vi "CH0_write_byte_data_into_mem_no_g_Rev01.vi"(0 "MB data":u8, 1 "UB data":u8, 3 "USB Interface Name":refnum<visa-resource-name>="COM3", 4 "HB data":u8, 5 "LB data":u8, 6 "MB address":string, 7 "HB address":string, 9 "WRITE DATA":bool, 10 "Input buffer size":u32=16384, 11 "LB address":string, 12 "UB address":string, 13 "error in (no error)":errorcluster) -> (14 "MB data string":string, 15 "UB data string":string, 17 "error out":errorcluster, 18 "HB data string":string, 19 "LB data string":string)   [LabVIEW 2012]
panel:
  out "T command Bytes sent 4":dbl
  out "T command Bytes sent 3":dbl
  out "T command Bytes sent 2":dbl
  out "T command Bytes sent":dbl
  out "First 'T' Number of bytes written":dbl
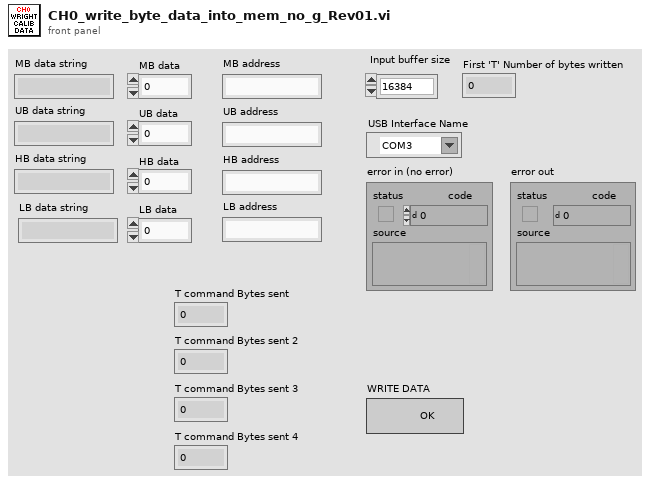
[diagram p1: front panel]
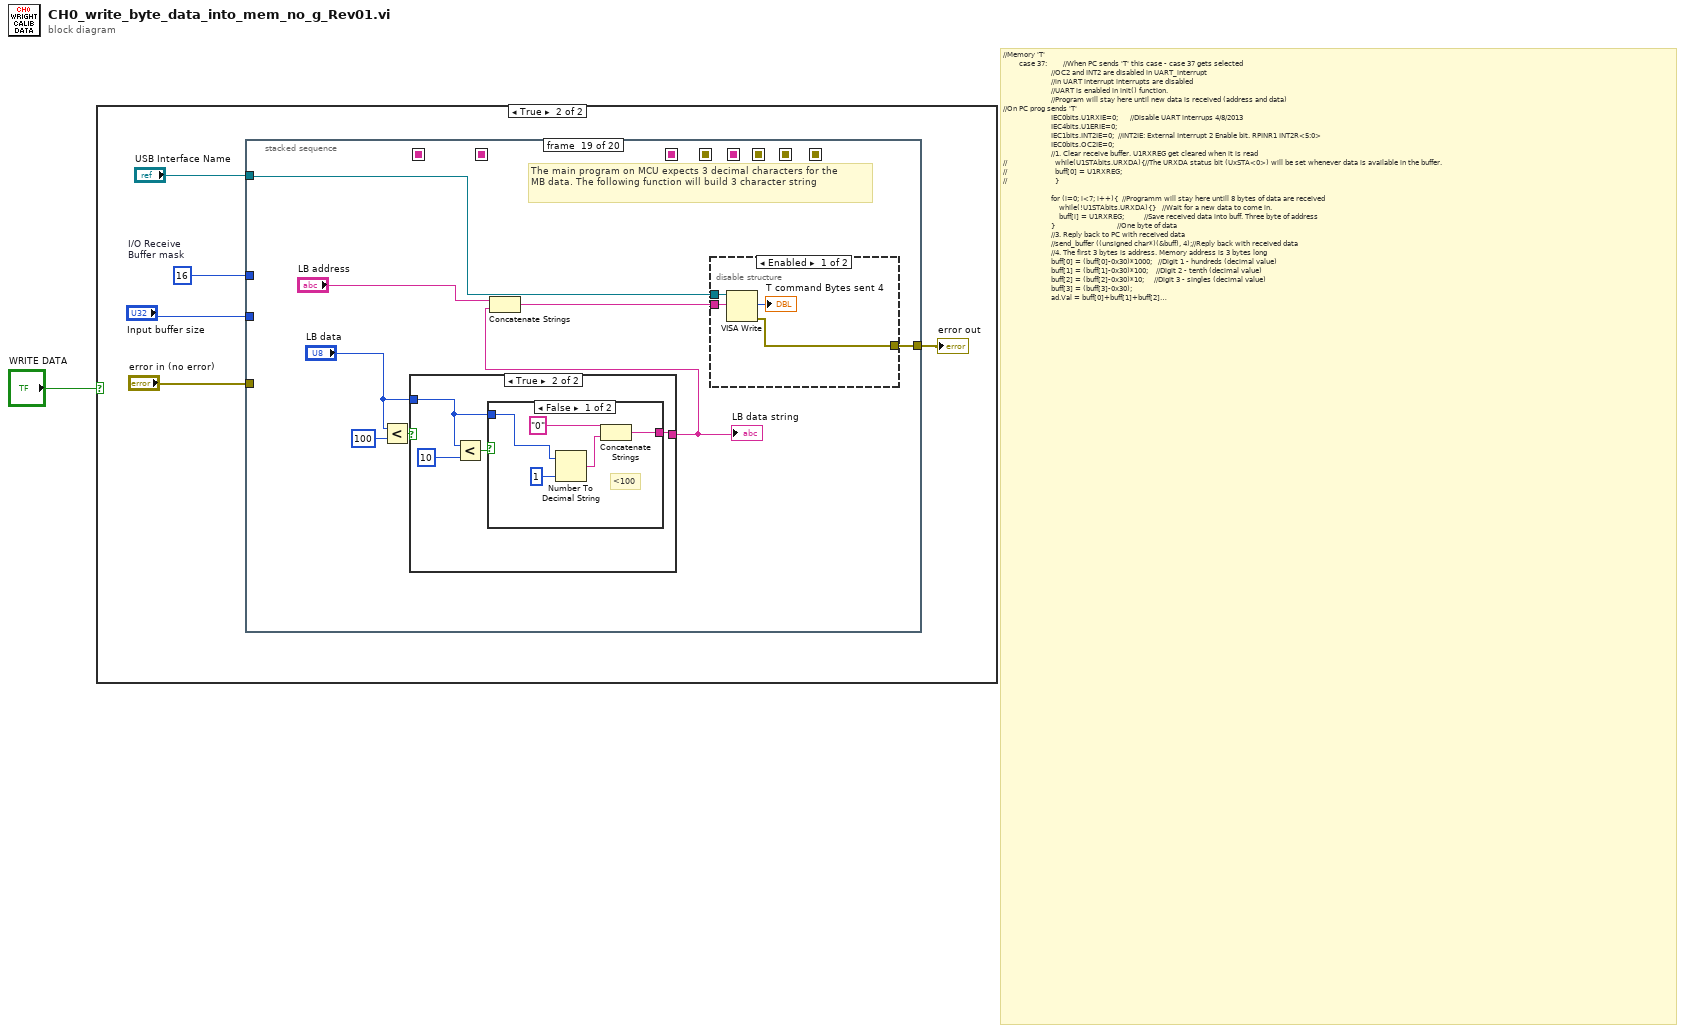
[diagram p0: block diagram]
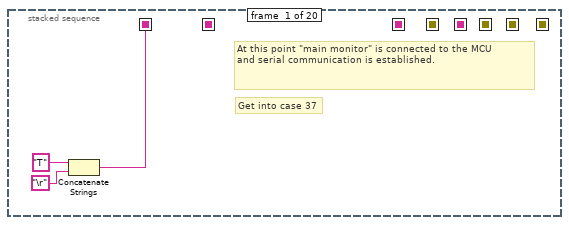
[diagram p3: hidden frame]
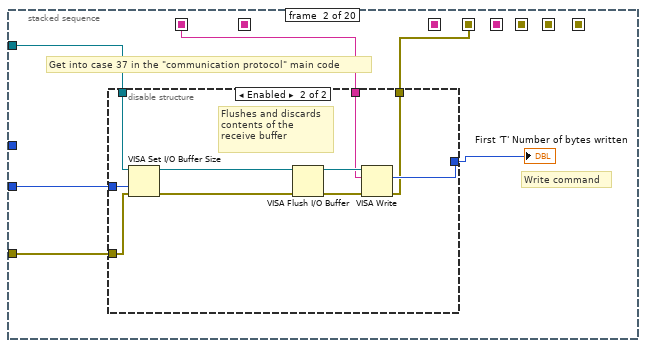
[diagram p4: hidden frame]
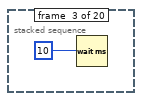
[diagram p6: hidden frame]
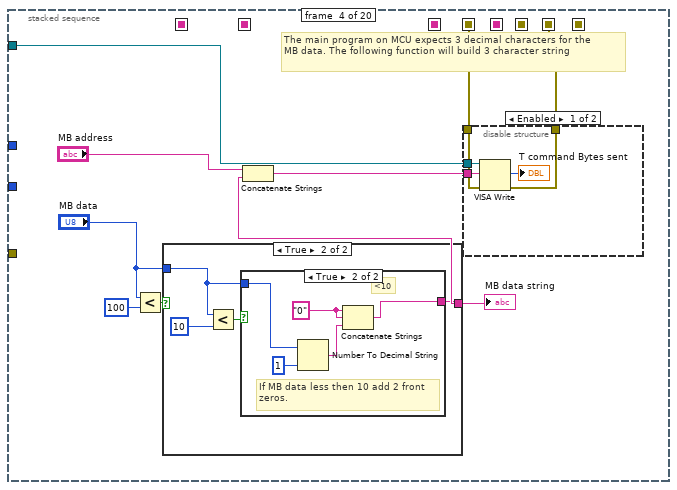
[diagram p7: hidden frame]
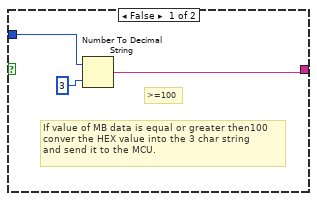
[diagram p8: hidden frame]
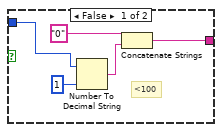
[diagram p9: hidden frame]
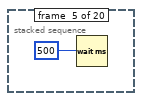
[diagram p11: hidden frame]
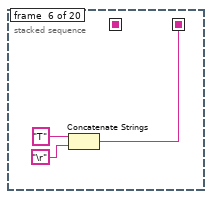
[diagram p12: hidden frame]
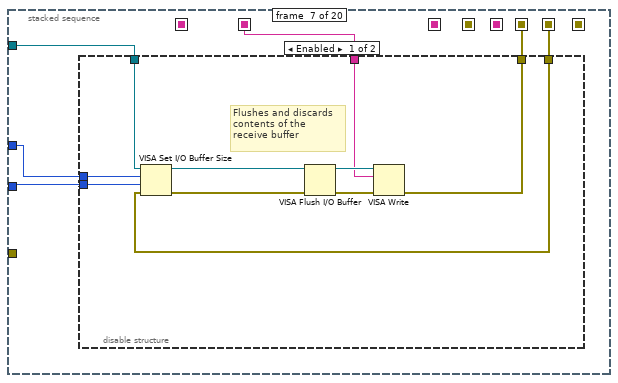
[diagram p13: hidden frame]
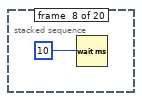
[diagram p15: hidden frame]
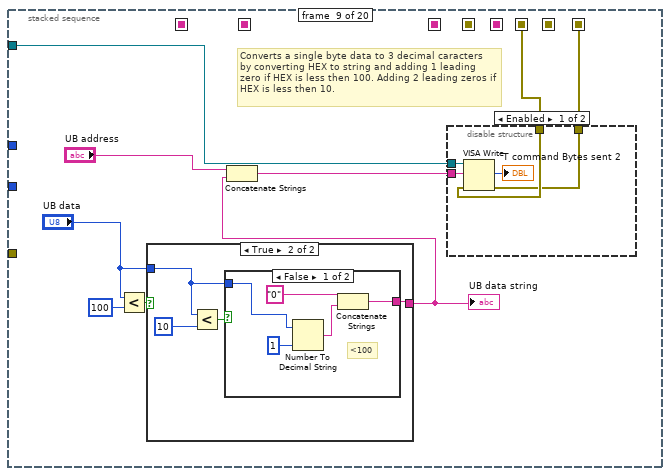
[diagram p16: hidden frame]
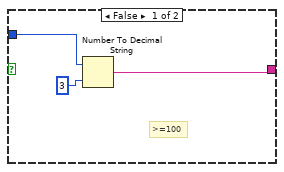
[diagram p17: hidden frame]
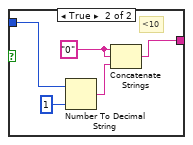
[diagram p18: hidden frame]
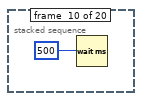
[diagram p20: hidden frame]
diagram:
  # "//Memory 'T'\n        case 37:        //When PC sends 'T' this case - case 37 gets selected\n                        //OC2 and INT2 are disabled in UART_interrupt\n                        //in UART interrupt interrupts are disabled\n                        //UART is enabled in init() function.\n                        //Program will stay here until new data is received (address and data)\n//On PC prog sends 'T'\n                        IEC0bits.U1RXIE=0;      //Disable UART interrups 4/8/2013\n                        IEC4bits.U1ERIE=0;\n                        IEC1bits.INT2IE=0;  //INT2IE: External Interrupt 2 Enable bit. RPINR1 INT2R<5:0>\n                        IEC0bits.OC2IE=0;\n                        //1. Clear receive buffer. U1RXREG get cleared when it is read\n//                        while(U1STAbits.URXDA){//The URXDA status bit (UxSTA<0>) will be set whenever data is available in the buffer.\n//                        buff[0] = U1RXREG;\n//                        }\n\n                        for (i=0; i<7; i++){  //Programm will stay here untill 8 bytes of data are received\n                            while(!U1STAbits.URXDA){}   //Wait for a new data to come in.\n                            buff[i] = U1RXREG;          //Save received data into buff. Three byte of address\n                        }                               //One byte of data\n                        //3. Reply back to PC with received data\n                        //send_buffer ((unsigned char*)(&buff), 4);//Reply back with received data\n                        //4. The first 3 bytes is address. Memory address is 3 bytes long\n                        buff[0] = (buff[0]-0x30)*1000;   //Digit 1 - hundreds (decimal value)\n                        buff[1] = (buff[1]-0x30)*100;    //Digit 2 - tenth (decimal value)\n                        buff[2] = (buff[2]-0x30)*10;     //Digit 3 - singles (decimal value)\n                        buff[3] = (buff[3]-0x30);\n                        ad.Val = buff[0]+buff[1]+buff[2]+buff[3];\n//                        send_char((char) ad.byte.MB);\n//                        send_char((char) ad.byte.UB);\n//                        send_char((char) ad.byte.HB);\n//                        send_char((char) ad.byte.LB); \n                        //5. The last 3 bytes are data\n                        buff[4] = buff[4]-0x30;//Load data. Byte number 4 is the data byte\n                        buff[5] = buff[5]-0x30;\n                        buff[6] = buff[6]-0x30;\n                        data = buff[4]*100+buff[5]*10+buff[6]; //Decimal value of 3 char digits\n                        //send_buffer ((unsigned char*)(&ad), 3);//Send back the received address\n                        //Erase byte by writing FFH into the address\n                        DF_WriteProtectDisable();   //Enable write to memory\n                        DF_IsBusy();                //Wait until the operation is done\n                        DF_WriteByte(ad.Val, data); //Write data into ad\n                        DF_IsBusy();\n                        DF_WriteDisable();          //Disable write\n                        DF_IsBusy();                        \n                        data=DF_ReadByte(ad.Val);     //4/22/13 return BYTE data\n//                       send_char((char) data);              //Read the memory location and reply with previously sent data\n//                        //Memory address for sign\n//                        buff[7] = (buff[7]-0x30)*1000;   //Digit 1 - hundreds (decimal value)\n//                        buff[8] = (buff[8]-0x30)*100;    //Digit 2 - tenth (decimal value)\n//                        buff[9] = (buff[9]-0x30)*10;     //Digit 3 - singles (decimal value)\n//                        buff[10] = (buff[10]-0x30);\n//                        ad.Val = buff[7]+buff[8]+buff[9]+buff[10];\n//                        //sign\n//                        sgn = buff[11];//<12\n                        \n                        selection = 1;\n                        rx_function=0; //4/11/13\n                        IEC0bits.U1RXIE=1;      //Reinable UART interrups\n                        IEC4bits.U1ERIE=1;                        \n                        IEC1bits.INT2IE=1;  //INT2IE: External Interrupt 2 Enable bit. RPINR1 INT2R<5:0>\n                        IEC0bits.OC2IE=1;\n                        \n\n            break;"
  n1 = case shown="True" "WRITE DATA" {
    frame False {
    }
    frame True {
      w4 = u16 16  # I/O Receive Buffer mask
      n2 = stacked-sequence {
        seq-local: [w7 _ _ _ _ _ _ _ _ _ _ _ _ _ _ _ _ _ _ _] -> [_ w12 _ _ _ _ _ _ _ _ _ _ _ _ _ _ _ _ _ _]
        seq-local: [_ _ _ _ _ w59 _ _ _ _ _ _ _ _ _ _ _ _ _ _] -> [_ _ _ _ _ _ w64 _ _ _ _ _ _ _ _ _ _ _ _ _]
        seq-local: [_ _ _ _ _ _ _ _ _ _ w111 _ _ _ _ _ _ _ _ _] -> [_ _ _ _ _ _ _ _ _ _ _ w115 _ _ _ _ _ _ _ _]
        seq-local: [_ _ _ _ _ _ _ _ _ _ _ _ _ _ _ w157 _ _ _ _] -> [_ _ _ _ _ _ _ _ _ _ _ _ _ _ _ _ w160 _ _ _]
        seq-local: [_ w10 _ _ _ _ _ _ _ _ _ _ _ _ _ _ _ _ _ _] -> [_ _ _ w28 _ _ _ _ _ _ _ _ _ _ _ _ _ _ _ _]
        seq-local: [_ _ _ w27 _ _ _ _ _ _ _ _ _ _ _ _ _ _ _ _] -> [_ _ _ _ _ _ w63 _ _ _ _ _ _ _ _ _ _ _ _ _]
        seq-local: [_ _ _ _ _ _ w62 _ _ _ _ _ _ _ _ _ _ _ _ _] -> [_ _ _ _ _ _ _ _ w80 _ _ _ _ _ _ _ _ _ _ _]
        seq-local: [_ _ _ _ _ _ _ _ w79 _ _ _ _ _ _ _ _ _ _ _] -> [_ _ _ _ _ _ _ _ _ _ _ w114 _ _ _ _ _ _ _ _]
        tunnel: "USB Interface Name" -> [_ w15 _ w34 _ _ w67 _ w82 _ _ w118 _ w130 _ _ w164 _ w178 _]
        tunnel: "error in (no error)" -> [_ w14 _ _ _ _ _ _ _ _ _ _ _ _ _ _ w162 _ _ _]
        tunnel: "Input buffer size" -> [_ w13 _ _ _ _ w66 _ _ _ _ w116 _ _ _ _ w163 _ _ _]
        tunnel: w4 -> [_ _ _ _ _ _ w65 _ _ _ _ w117 _ _ _ _ w161 _ _ _]
        tunnel: [_ _ _ _ _ _ _ _ _ _ _ _ _ _ _ _ _ _ w176 _] -> w3
        frame #0 {
          # "At this point \"main monitor\" is connected to the MCU\nand serial communication is established."
          # "Get into case 37"
          n3 = Concatenate Strings("T", "\r") -> (w7:string)
        }
        frame #1 {
          # "Get into case 37 in the \"communication protocol\" main code"
          # "Write command"
          n4 = disable-structure shown="Enabled" {
            disable-tunnel: w13 -> [_ w21]
            disable-tunnel: w12 -> [_ w20]
            disable-tunnel: w15 -> [_ w19]
            disable-tunnel: w14 -> [_ w18]
            disable-tunnel: [_ w17] -> w11
            disable-tunnel: [_ w16] -> w10
            frame Disabled {
            }
            frame Enabled {
              # "Flushes and discards \ncontents of the \nreceive buffer"
              n5 = VISA Set I/O Buffer Size(VISA resource name=w19, size (4096)=w21, error in (no error)=w18) -> (VISA resource name out=w23:refnum<visa-resource-name>, error out=w22:errorcluster)  [unwired: 1 in]
              n6 = VISA Flush I/O Buffer(VISA resource name=w23, error in (no error)=w22) -> (VISA resource name out=w25:refnum<visa-resource-name>, error out=w24:errorcluster)  [unwired: 1 in]
              n7 = VISA Write(VISA resource name=w25, write buffer=w20, error in (no error)=w24) -> (return count=w17:u32, error out=w16:errorcluster)  [unwired: 1 out]
            }
          }
          "First 'T' Number of bytes written" <- w11
        }
        frame #2 {
          n8 = Wait (ms)(milliseconds to wait=10) -> ()  [unwired: 1 out]
        }
        frame #3 {
          # "The main program on MCU expects 3 decimal characters for the \nMB data. The following function will build 3 character string"
          n9 = Less?(x="MB data", y=100) -> (x < y?=w32:bool)
          n10 = case shown="True" w32 {
            tunnel: [w38 w39] -> w29
            tunnel: "MB data" -> [w36 w40]
            frame False {
              # "If value of MB data is equal or greater then100\nconver the HEX value into the 3 char string \nand send it to the MCU."
              # ">=100"
              n11 = Number To Decimal String(number=w36, width (-)=3) -> (decimal integer string=w38:string)
            }
            frame True {
              n12 = Less?(x=w40, y=10) -> (x < y?=w42:bool)
              n13 = case shown="True" w42 {
                tunnel: w40 -> [w44 w48]
                tunnel: [w43 w49] -> w39
                frame False {
                  # "<100"
                  n14 = Number To Decimal String(number=w44, width (-)=1) -> (decimal integer string=w45:string)
                  n15 = Concatenate Strings("0", w45) -> (w43:string)
                }
                frame True {
                  w50 = "0"
                  # "If MB data less then 10 add 2 front\nzeros."
                  # "<10"
                  n16 = Number To Decimal String(number=w48, width (-)=1) -> (decimal integer string=w51:string)
                  n17 = Concatenate Strings(w50, w50, w51) -> (w49:string)
                }
              }
            }
          }
          "MB data string" <- w29
          n18 = Concatenate Strings("MB address", w29) -> (w35:string)
          n19 = disable-structure shown="Enabled" {
            disable-tunnel: w35 -> [w56 _]
            disable-tunnel: w34 -> [w55 _]
            disable-tunnel: w28 -> [w54 _]
            disable-tunnel: [w53 _] -> w27
            frame Enabled {
              n20 = VISA Write(VISA resource name=w55, write buffer=w56, error in (no error)=w54) -> (return count=→"T command Bytes sent":u32, error out=w53:errorcluster)  [unwired: 1 out]
            }
            frame Disabled {
            }
          }
        }
        frame #4 {
          n21 = Wait (ms)(milliseconds to wait=500) -> ()  [unwired: 1 out]
        }
        frame #5 {
          n22 = Concatenate Strings("T", "\r") -> (w59:string)
        }
        frame #6 {
          n23 = disable-structure shown="Enabled" {
            disable-tunnel: w67 -> [w73 _]
            disable-tunnel: w66 -> [w72 _]
            disable-tunnel: w65 -> [w71 _]
            disable-tunnel: w64 -> [w70 _]
            disable-tunnel: w63 -> [w69 _]
            disable-tunnel: [w68 _] -> w62
            frame Enabled {
              # "Flushes and discards \ncontents of the \nreceive buffer"
              n24 = VISA Set I/O Buffer Size(VISA resource name=w73, mask (16)=w71, size (4096)=w72, error in (no error)=w69) -> (VISA resource name out=w75:refnum<visa-resource-name>, error out=w74:errorcluster)
              n25 = VISA Flush I/O Buffer(VISA resource name=w75, error in (no error)=w74) -> (VISA resource name out=w77:refnum<visa-resource-name>, error out=w76:errorcluster)  [unwired: 1 in]
              n26 = VISA Write(VISA resource name=w77, write buffer=w70, error in (no error)=w76) -> (error out=w68:errorcluster)  [unwired: 2 out]
            }
            frame Disabled {
            }
          }
        }
        frame #7 {
          n27 = Wait (ms)(milliseconds to wait=10) -> ()  [unwired: 1 out]
        }
        frame #8 {
          # "Converts a single byte data to 3 decimal caracters\nby converting HEX to string and adding 1 leading zero if HEX is less then 100. Adding 2 leading zeros if HEX is less then 10."
          n28 = Less?(x="UB data", y=100) -> (x < y?=w86:bool)
          n29 = case shown="True" w86 {
            tunnel: [w90 w91] -> w83
            tunnel: "UB data" -> [w88 w92]
            frame False {
              # ">=100"
              n30 = Number To Decimal String(number=w88, width (-)=3) -> (decimal integer string=w90:string)
            }
            frame True {
              n31 = Less?(x=w92, y=10) -> (x < y?=w94:bool)
              n32 = case shown="False" w94 {
                tunnel: w92 -> [w96 w100]
                tunnel: [w95 w101] -> w91
                frame False {
                  # "<100"
                  n33 = Number To Decimal String(number=w96, width (-)=1) -> (decimal integer string=w97:string)
                  n34 = Concatenate Strings("0", w97) -> (w95:string)
                }
                frame True {
                  w102 = "0"
                  # "<10"
                  n35 = Number To Decimal String(number=w100, width (-)=1) -> (decimal integer string=w103:string)
                  n36 = Concatenate Strings(w102, w102, w103) -> (w101:string)
                }
              }
            }
          }
          "UB data string" <- w83
          n37 = Concatenate Strings("UB address", w83) -> (w87:string)
          n38 = disable-structure shown="Enabled" {
            disable-tunnel: w87 -> [w108 _]
            disable-tunnel: w82 -> [w107 _]
            disable-tunnel: w80 -> [w106 _]
            disable-tunnel: [w105 _] -> w79
            frame Enabled {
              n39 = VISA Write(VISA resource name=w107, write buffer=w108, error in (no error)=w106) -> (return count=→"T command Bytes sent 2":u32, error out=w105:errorcluster)  [unwired: 1 out]
            }
            frame Disabled {
            }
          }
        }
        frame #9 {
          n40 = Wait (ms)(milliseconds to wait=500) -> ()  [unwired: 1 out]
        }
        frame #10 {
          n41 = Concatenate Strings("T", "\r") -> (w111:string)
        }
        frame #11 {
          n42 = disable-structure shown="Enabled" {
            disable-tunnel: w118 -> [w123 _]
            disable-tunnel: w117 -> [w122 _]
            disable-tunnel: w116 -> [w121 _]
            disable-tunnel: w115 -> [w120 _]
            disable-tunnel: w114 -> [w119 _]
            frame Enabled {
              # "Flushes and discards \ncontents of the \nreceive buffer"
              n43 = VISA Set I/O Buffer Size(VISA resource name=w123, mask (16)=w122, size (4096)=w121, error in (no error)=w119) -> (VISA resource name out=w125:refnum<visa-resource-name>, error out=w124:errorcluster)
              n44 = VISA Flush I/O Buffer(VISA resource name=w125, error in (no error)=w124) -> (VISA resource name out=w127:refnum<visa-resource-name>, error out=w126:errorcluster)  [unwired: 1 in]
              n45 = VISA Write(VISA resource name=w127, write buffer=w120, error in (no error)=w126) -> ()  [unwired: 3 out]
            }
            frame Disabled {
            }
          }
        }
        frame #12 {
          n46 = Wait (ms)(milliseconds to wait=10) -> ()  [unwired: 1 out]
        }
        frame #13 {
          # "Converts a single byte data to 3 decimal caracters\nby converting HEX to string and adding 1 leading zero if HEX is less then 100. Adding 2 leading zeros if HEX is less then 10."
          n47 = Less?(x="HB data", y=100) -> (x < y?=w134:bool)
          n48 = case shown="True" w134 {
            tunnel: [w138 w139] -> w131
            tunnel: "HB data" -> [w136 w140]
            frame False {
              # ">=100"
              n49 = Number To Decimal String(number=w136, width (-)=3) -> (decimal integer string=w138:string)
            }
            frame True {
              n50 = Less?(x=w140, y=10) -> (x < y?=w142:bool)
              n51 = case shown="False" w142 {
                tunnel: w140 -> [w144 w148]
                tunnel: [w143 w149] -> w139
                frame False {
                  # "<100"
                  n52 = Number To Decimal String(number=w144, width (-)=1) -> (decimal integer string=w145:string)
                  n53 = Concatenate Strings("0", w145) -> (w143:string)
                }
                frame True {
                  w150 = "0"
                  # "<10"
                  n54 = Number To Decimal String(number=w148, width (-)=1) -> (decimal integer string=w151:string)
                  n55 = Concatenate Strings(w150, w150, w151) -> (w149:string)
                }
              }
            }
          }
          "HB data string" <- w131
          n56 = Concatenate Strings("HB address", w131) -> (w135:string)
          n57 = disable-structure shown="Enabled" {
            disable-tunnel: w135 -> [w154 _]
            disable-tunnel: w130 -> [w153 _]
            frame Enabled {
              n58 = VISA Write(VISA resource name=w153, write buffer=w154) -> (return count=→"T command Bytes sent 3":u32)  [unwired: 1 in, 2 out]
            }
            frame Disabled {
            }
          }
        }
        frame #14 {
          n59 = Wait (ms)(milliseconds to wait=500) -> ()  [unwired: 1 out]
        }
        frame #15 {
          # "Get into case 37"
          n60 = Concatenate Strings("T", "\r") -> (w157:string)
        }
        frame #16 {
          # "Get into case 37 in the communication protocol"
          # "Write command"
          n61 = disable-structure shown="Enabled" {
            disable-tunnel: w163 -> [w170 _]
            disable-tunnel: w160 -> [w169 _]
            disable-tunnel: w164 -> [w168 _]
            disable-tunnel: w162 -> [w167 _]
            disable-tunnel: [w166 _] -> _
            disable-tunnel: w161 -> [w165 _]
            frame Enabled {
              # "Flushes and discards \ncontents of the \nreceive buffer"
              n62 = VISA Set I/O Buffer Size(VISA resource name=w168, mask (16)=w165, size (4096)=w170, error in (no error)=w167) -> (VISA resource name out=w172:refnum<visa-resource-name>, error out=w171:errorcluster)
              n63 = VISA Flush I/O Buffer(VISA resource name=w172, error in (no error)=w171) -> (VISA resource name out=w174:refnum<visa-resource-name>, error out=w173:errorcluster)  [unwired: 1 in]
              n64 = VISA Write(VISA resource name=w174, write buffer=w169, error in (no error)=w173) -> (return count=w166:u32)  [unwired: 2 out]
            }
            frame Disabled {
            }
          }
        }
        frame #17 {
          n65 = Wait (ms)(milliseconds to wait=10) -> ()  [unwired: 1 out]
        }
        frame #18 {
          # "The main program on MCU expects 3 decimal characters for the \nMB data. The following function will build 3 character string"
          n66 = Less?(x="LB data", y=100) -> (x < y?=w182:bool)
          n67 = case shown="True" w182 {
            tunnel: [w186 w187] -> w179
            tunnel: "LB data" -> [w184 w188]
            frame False {
              # ">=100"
              n68 = Number To Decimal String(number=w184, width (-)=3) -> (decimal integer string=w186:string)
            }
            frame True {
              n69 = Less?(x=w188, y=10) -> (x < y?=w190:bool)
              n70 = case shown="False" w190 {
                tunnel: w188 -> [w192 w196]
                tunnel: [w191 w197] -> w187
                frame False {
                  # "<100"
                  n71 = Number To Decimal String(number=w192, width (-)=1) -> (decimal integer string=w193:string)
                  n72 = Concatenate Strings("0", w193) -> (w191:string)
                }
                frame True {
                  w198 = "0"
                  # "<10"
                  n73 = Number To Decimal String(number=w196, width (-)=1) -> (decimal integer string=w199:string)
                  n74 = Concatenate Strings(w198, w198, w199) -> (w197:string)
                }
              }
            }
          }
          "LB data string" <- w179
          n75 = Concatenate Strings("LB address", w179) -> (w183:string)
          n76 = disable-structure shown="Enabled" {
            disable-tunnel: w183 -> [w203 _]
            disable-tunnel: w178 -> [w202 _]
            disable-tunnel: [w201 _] -> w176
            frame Enabled {
              n77 = VISA Write(VISA resource name=w202, write buffer=w203) -> (return count=→"T command Bytes sent 4":u32, error out=w201:errorcluster)  [unwired: 1 in, 1 out]
            }
            frame Disabled {
            }
          }
        }
        frame #19 {
          n78 = Wait (ms)(milliseconds to wait=500) -> ()  [unwired: 1 out]
        }
      }
      "error out" <- w3
    }
  }
